vi "Apply Transformations.vi"(8 "error in (no error)":errorcluster, 11 "Tool Path in":refnum<class "Tool Path.lvclass">) -> (0 "error out":errorcluster, 3 "Tool Path out":refnum<class "Tool Path.lvclass">)   [LabVIEW 2019, in "Tool Path.lvclass"]
uses:
  Tool Path.lvclass
  Parse/ParsePaths/Path.lvclass/Path.ctl
  Parse/PathCommands/Point.ctl
  Parse/Transform/Transform.lvclass/Transform.ctl
  <vilib>/Analysis/baseanly.llb/Real A x B.vi
  Parse/PathCommands/PathCommands.lvclass
  Parse/Transform/Transform.lvclass
  Parse/ParsePaths/Path.lvclass
  <vilib>/Analysis/NI_AALBase.lvlib
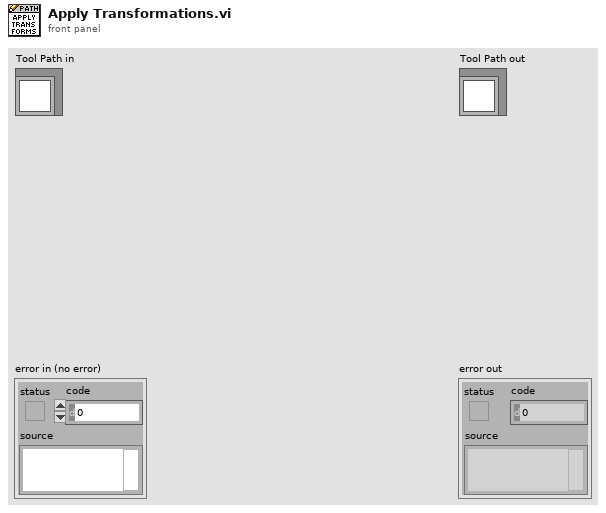
[diagram p1: front panel]
types:
  T1 = typedef "PathCommands.lvclass/Point.ctl" = cluster{"X":dbl, "Y":dbl}
  T2 = typedef "NI_Matrix.lvlib/RealMatrix.ctl" = dbl[][]
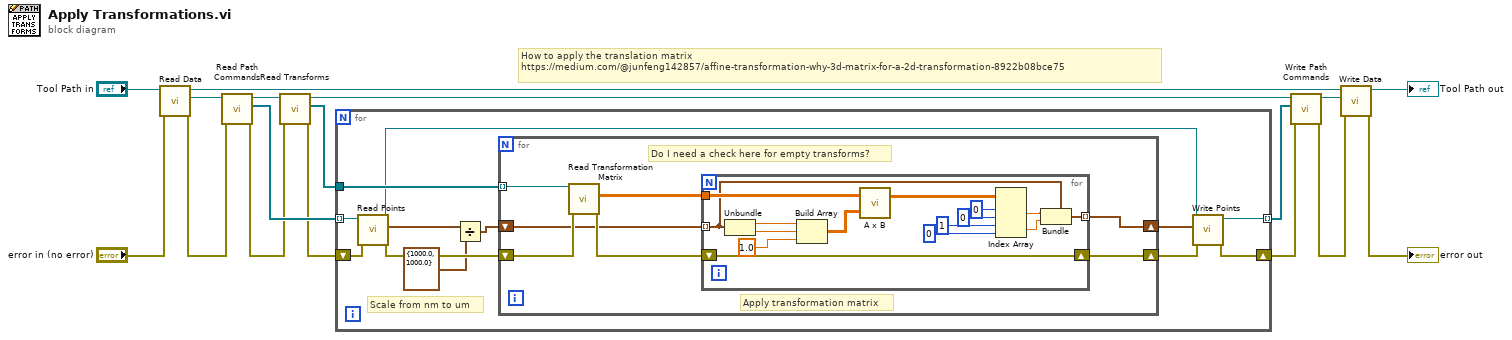
[diagram p0: block diagram]
diagram:
  # "How to apply the translation matrix\nhttps://medium.com/@junfeng142857/affine-transformation-why-3d-matrix-for-a-2d-transformation-8922b08bce75"
  n1 = call-dynamic "Read Data.vi"("error in (no error)"="error in (no error)", "Tool Path in"="Tool Path in") -> ("error out"=w1:errorcluster, "Path.lvclass"=w8:refnum<class "Path.lvclass">, "Tool Path out"=w7:refnum<class "Tool Path.lvclass">)  [unwired: 7 in]
  n2 = call "Read Path Commands.vi"("error in (no error)"=w1, "Path in"=w8) -> ("error out"=w13:errorcluster, "Path Commands"=w16:refnum<class "PathCommands.lvclass">[], "Path out"=w17:refnum<class "Path.lvclass">)  [unwired: 7 in]
  n3 = call "Read Transforms.vi"("error in (no error)"=w13, "Path in"=w17) -> ("error out"=w14:errorcluster, "Transforms"=w15:refnum<class "Transform.lvclass">[], "Path out"=w11:refnum<class "Path.lvclass">)  [unwired: 7 in]
  n4 = for {
    shift-right: [w24] -> w10
    shift-left: w14 -> [w29]
    tunnel: w16 -> [w28] mode=indexing
    tunnel: w15 -> [w27]
    tunnel: [w21] -> w12 mode=indexing
    # "Scale from nm to um"
    n5 = call-dynamic "Read Points.vi"("error in (no error)"=w29, "PathCommands in"=w28) -> ("error out"=w23:errorcluster, "Points"=w19:T1[], "PathCommands out"=w25:refnum<class "PathCommands.lvclass">)  [unwired: 7 in]
    n6 = Divide(x=w19, y=T1 {"X"=1000.0, "Y"=1000.0} ("Point")) -> (x/y=w18:T1[])
    n7 = for {
      tunnel: w27 -> [w36] mode=indexing
      shift-right: [w34] -> w26
      shift-left: w18 -> [w30]
      shift-right: [w33] -> w22
      shift-left: w23 -> [w32]
      # "Apply transformation matrix"
      # "Do I need a check here for empty transforms?"
      n8 = call "Read Transformation Matrix.vi"("error in (no error)"=w32, "Transform in"=w36) -> ("error out"=w31:errorcluster, "Real Matrix"=w35:T2)  [unwired: 7 in, 1 out]
      n9 = for {
        tunnel: w35 -> [w49]
        tunnel: w30 -> [w42] mode=indexing
        tunnel: [w41] -> w34 mode=indexing
        shift-right: [w38] -> w33
        shift-left: w31 -> [w38]
        n10 = Unbundle(w42) -> ("X"=w51:dbl, "Y"=w50:dbl)
        n11 = Build Array(w51, w50, 1.0) -> (w37:T2)
        n12 = call-poly <vilib>:"A x B.vi"("B"=w37, "A"=w49) -> ("A x B"=w48:T2)  [unwired: 1 out]
        n13 = Index Array(array=w48, index (row) #1=0 ("index (row)"), index (col) #1=0 ("index (col)"), index (row) #2=1 ("index (row)"), index (col) #2=0 ("index (col)")) -> (element #1=w44:dbl, element #2=w43:dbl)
        n14 = Bundle(cluster=w42, "X"=w44, "Y"=w43) -> (w41:T1)
      }
    }
    n15 = call-dynamic "Write Points.vi"("error in (no error)"=w22, "Points"=w26, "PathCommands in"=w25) -> ("error out"=w24:errorcluster, "PathCommands out"=w21:refnum<class "PathCommands.lvclass">)  [unwired: 7 in]
  }
  n16 = call "Write Path Commands.vi"("error in (no error)"=w10, "Path Commands"=w12, "Path in"=w11) -> ("error out"=w5:errorcluster, "Path out"=w6:refnum<class "Path.lvclass">)  [unwired: 7 in]
  n17 = call-dynamic "Write Data.vi"("error in (no error)"=w5, "Path.lvclass"=w6, "Tool Path in"=w7) -> ("error out"=→"error out":errorcluster, "Tool Path out"=→"Tool Path out":refnum<class "Tool Path.lvclass">)  [unwired: 7 in]
